vi "Validate Lens B.vi"(2 "Error In":errorcluster, 3 "Units":bool, 4 "Parameters In":T1 {"RunType" items=["Diagnostics", "Tune", "Acquisition"]}, 5 "Lenses":T5[](array[typedef])) -> (0 "Error Out":errorcluster, 1 "Lens Table":string[][](table))   [LabVIEW 2018]
uses:
  Type Defs/Lenses.ctl
  Type Defs/Global Configrations.ctl
  Type Defs/Configration.ctl
  GC-MSMSDevlopment/Type/_RT Configuration 2.ctl
  Type Defs/ADC Table.ctl
  Type Defs/Global Action.ctl
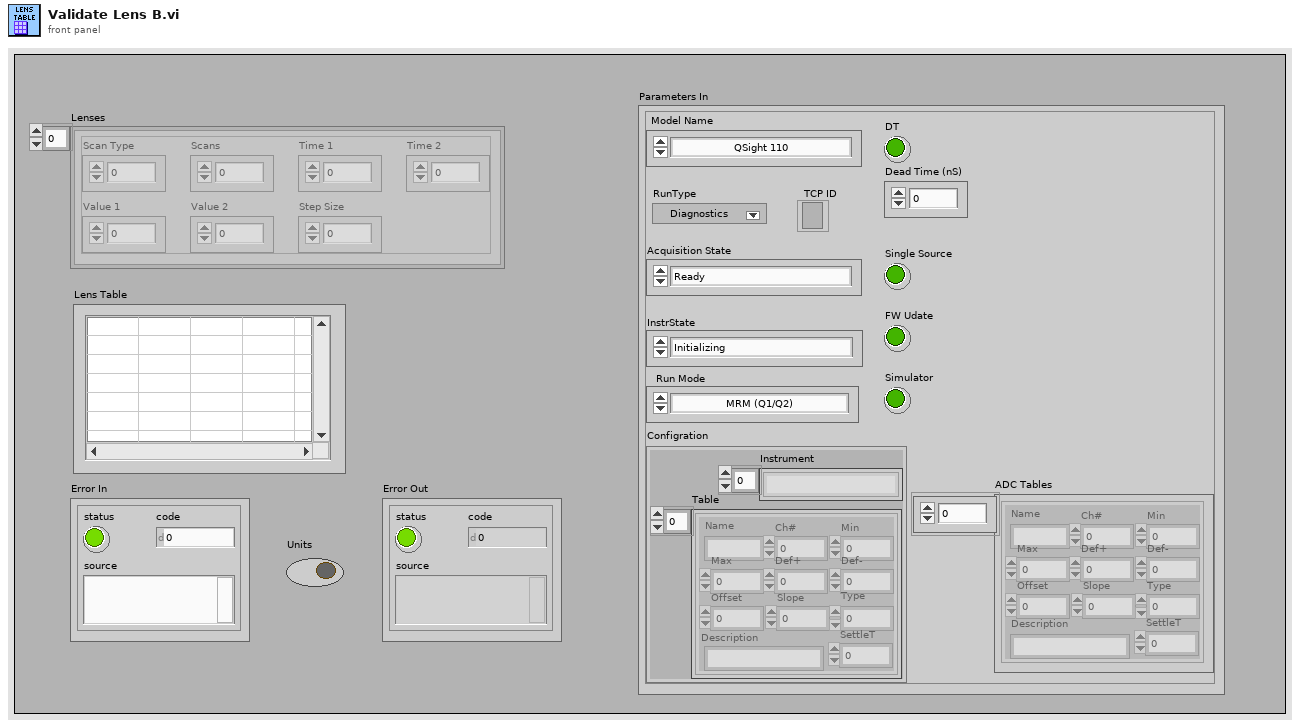
[diagram p1: front panel]
types:
  T1 = typedef "Global Configrations.ctl" = cluster{"Model Name":enum16{"QSight 110", "QSight 120", "QSight 210", "QSight 220", "QSight 410", "QSight 420", "IONICS 3Q 110", "IONICS 3Q 120", "IONICS 3Q 210", "IONICS 3Q 220", "IONICS 3Q 310", "IONICS 3Q 320", "Simulation (Single Source)", "Simulation (Dual Source)"}, "RunType":u16, "Acquisition State":enum16{"Ready", "Busy", "Waiting"}, "InstrState":enum16{"Initializing", "Mass Spectrometer is Off", "Starting Up", "Turning Power Off", "Going to Standby", "Roughing Pump Ready", "Turning Turbo Off", "Turbo Startup", "Turbopump Ready", "Checking Vacuum", "Going to Ready", "Ready", "Running", "Source Standby", "Lost Communication", "Shutting Down", "Fault", "24V Standby", "Go to 24V Standby", "Turbopump Ready-Waiting"}, "Run Mode":enum16{"MRM (Q1/Q2)", "Q1 Scan", "Q1 SRM", "Q2 Scan", "Q2 SRM", "Product Scan", "Precursor Scan", "Neutral Loss", "Neutral Gain"}, "Configration":T2, "TCP ID":refnum<k5>, "DT":bool, "Dead Time (nS)":i32, "Single Source":bool, "ADC Tables":T4[], "FW Udate":bool, "Simulator":bool}
  T2 = typedef "Configration.ctl" = cluster{"Table":T3[], "Instrument":string[]}
  T3 = typedef "_RT Configuration 2.ctl" = cluster{"Name":string, "Ch#":u8, "Min":dbl, "Max":dbl, "Def+":dbl, "Def-":dbl, "Offset":dbl, "Slope":dbl, "Type":u8, "Description":string, "SettleT":dbl}
  T4 = typedef "ADC Table.ctl" = cluster{"Name":string, "Ch#":u8, "Min":dbl, "Max":dbl, "Def+":dbl, "Def-":dbl, "Offset":dbl, "Slope":dbl, "Type":u8, "Description":string, "SettleT":dbl}
  T5 = typedef "Lenses.ctl" = cluster{"Scan Type":u8, "Scans":i32, "Time 1":dbl, "Time 2":dbl, "Value 1":dbl, "Value 2":dbl, "Step Size":dbl}
  T6 = typedef "Global Action.ctl" = enum16{"Write", "Read"}
  T7 = typedef "Global Parameters.ctl" = cluster{"Calibrations":cluster{"Q1 +ve":dbl[][], "Q2 +ve":dbl[][], "Q1 -ve":dbl[][], "Q2 -ve":dbl[][]}, "Resolution Q1":cluster{"High +ve":dbl[][], "Med +ve":dbl[][], "Low +ve":dbl[][], "High -ve":dbl[][], "Med -ve":dbl[][], "Low -ve":dbl[][]}, "Resolution Q2":cluster{"High +ve":dbl[][], "Med +ve":dbl[][], "Loe +ve":dbl[][], "High -ve":dbl[][], "Med -ve":dbl[][], "Low -ve":dbl[][]}, "MR Parameters":T8, "Mass":dbl[][], "Dwell":dbl[][], "Steps":i32[][], "Method Refnum":refnum<vi>}
  T8 = typedef "MR Parameters.ctl" = cluster{"Name":string, "Ch#":u8, "StartV":dbl, "StopV":dbl, "StepV":dbl, "Index":u8}
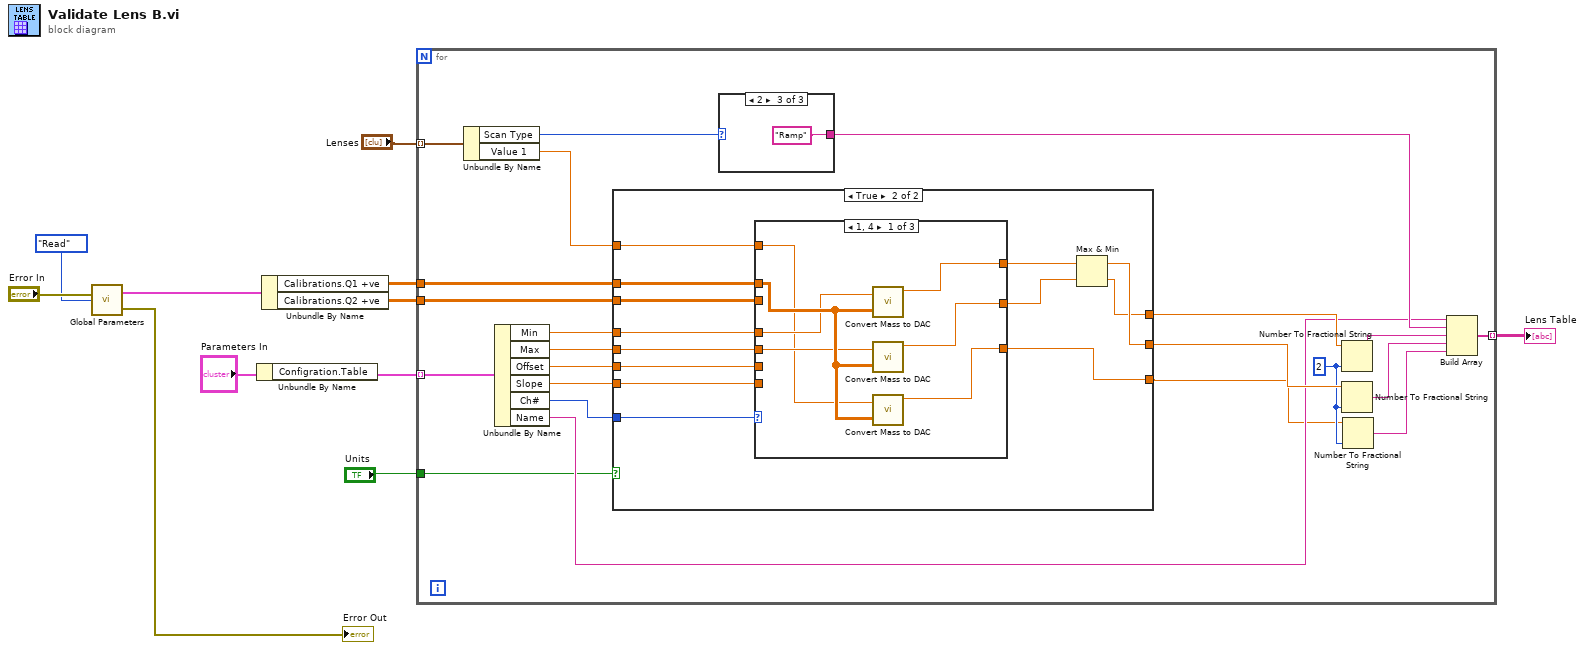
[diagram p0: block diagram]
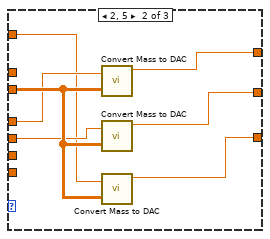
[diagram p3: hidden frame]
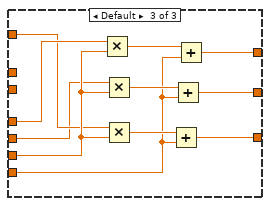
[diagram p4: hidden frame]
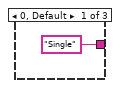
[diagram p5: hidden frame]
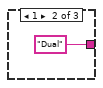
[diagram p6: hidden frame]
diagram:
  n1 = call "Global Parameters.vi"("Error In"="Error In", "Action"=Global_Action."Read") -> ("Error Out"=→"Error Out":errorcluster, "Parameters Out"=w10:T7)  [unwired: 1 in]
  n2 = Unbundle By Name("Parameters In") -> ("Configration.Table"=w2:T3[])
  n3 = Unbundle By Name(w10) -> ("Calibrations.Q1 +ve"=w9:dbl[][], "Calibrations.Q2 +ve"=w8:dbl[][])
  n4 = for {
    tunnel: "Lenses" -> [w26] mode=indexing
    tunnel: [w30] -> w7 mode=indexing
    tunnel: w2 -> [w27] mode=indexing
    tunnel: w9 -> [w20]
    tunnel: w8 -> [w19]
    tunnel: "Units" -> [w12]
    w23 = 2
    n5 = Unbundle By Name(w26) -> ("Scan Type"=w24:u8, "Value 1"=w25:dbl)
    n6 = Unbundle By Name(w27) -> ("Min"=w16:dbl, "Max"=w33:dbl, "Offset"=w15:dbl, "Slope"=w14:dbl, "Ch#"=w18:u8, "Name"=w17:string)
    n7 = case shown="True" w12 {
      tunnel: w33 -> [w36 w49]
      tunnel: [w35 w47] -> w31
      tunnel: [w36 w48] -> w32
      tunnel: w25 -> [w34 w46]
      tunnel: w18 -> [_ w45]
      tunnel: w20 -> [_ w44]
      tunnel: w19 -> [_ w43]
      tunnel: w16 -> [w35 w40]
      tunnel: w15 -> [_ w42]
      tunnel: w14 -> [_ w41]
      tunnel: [w34 w37] -> w13
      frame False {
      }
      frame True {
        n8 = case shown="1, 4" w45 {
          tunnel: w49 -> [w51 w61 w68]
          tunnel: w46 -> [w50 w60 w69]
          tunnel: w44 -> [w56 _ _]
          tunnel: w43 -> [_ w63 _]
          tunnel: w42 -> [_ _ w70]
          tunnel: w41 -> [_ _ w64]
          tunnel: w40 -> [w55 w62 w71]
          tunnel: [w52 w57 w67] -> w37
          tunnel: [w53 w58 w66] -> w38
          tunnel: [w54 w59 w65] -> w39
          frame 1, 4 {
            n9 = call "Convert Mass to DAC.vi"("Mass"=w55, "Calibration Table"=w56) -> ("DAC Value"=w54:dbl)  [unwired: 3 out]
            n10 = call "Convert Mass to DAC.vi"("Mass"=w51, "Calibration Table"=w56) -> ("DAC Value"=w53:dbl)  [unwired: 3 out]
            n11 = call "Convert Mass to DAC.vi"("Mass"=w50, "Calibration Table"=w56) -> ("DAC Value"=w52:dbl)  [unwired: 3 out]
          }
          frame 2, 5 {
            n12 = call "Convert Mass to DAC.vi"("Mass"=w62, "Calibration Table"=w63) -> ("DAC Value"=w59:dbl)  [unwired: 3 out]
            n13 = call "Convert Mass to DAC.vi"("Mass"=w61, "Calibration Table"=w63) -> ("DAC Value"=w58:dbl)  [unwired: 3 out]
            n14 = call "Convert Mass to DAC.vi"("Mass"=w60, "Calibration Table"=w63) -> ("DAC Value"=w57:dbl)  [unwired: 3 out]
          }
          frame Default {
            n15 = Multiply(x=w71, y=w70) -> (x*y=w74:dbl)
            n16 = Multiply(x=w68, y=w70) -> (x*y=w73:dbl)
            n17 = Multiply(x=w69, y=w70) -> (x*y=w72:dbl)
            n18 = Add(x=w72, y=w64) -> (x+y=w67:dbl)
            n19 = Add(x=w73, y=w64) -> (x+y=w66:dbl)
            n20 = Add(x=w74, y=w64) -> (x+y=w65:dbl)
          }
        }
        n21 = Max & Min(x=w39, y=w38) -> (max(x,y)=w48:dbl, min(x,y)=w47:dbl)
      }
    }
    n22 = case shown="2" w24 {
      tunnel: ["Single" ("Scan Type") "Dual" ("Scan Type") "Ramp" ("Scan Type")] -> w22
      frame 0, Default {
      }
      frame 1 {
      }
      frame 2 {
      }
    }
    n23 = Number To Fractional String(number=w31, precision (6)=w23) -> (F-format string=w21:string)  [unwired: 2 out]
    n24 = Number To Fractional String(number=w32, precision (6)=w23) -> (F-format string=w29:string)  [unwired: 2 out]
    n25 = Number To Fractional String(number=w13, precision (6)=w23) -> (F-format string=w28:string)  [unwired: 2 out]
    n26 = Build Array(w17, w22, w21, w29, w28) -> (w30:string[])
  }
  "Lens Table" <- w7
